vi "DAQNavi Create Channel(Buffered-CI-UpDown Count Value).vi"(0 "task in":i32=-1, 5 "physical channels":string="PCI-1784,BID#0/cntr0", 7 "signal counting type":string(combo)="PulseDirection", 11 "error in (no error)":errorcluster) -> (4 "task out":i32, 15 "error out":errorcluster)   [LabVIEW 2020]
uses:
  DAQNavi_LV.dll
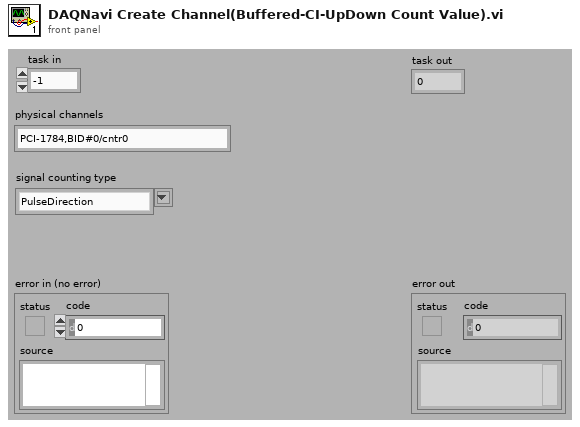
[diagram p1: front panel]
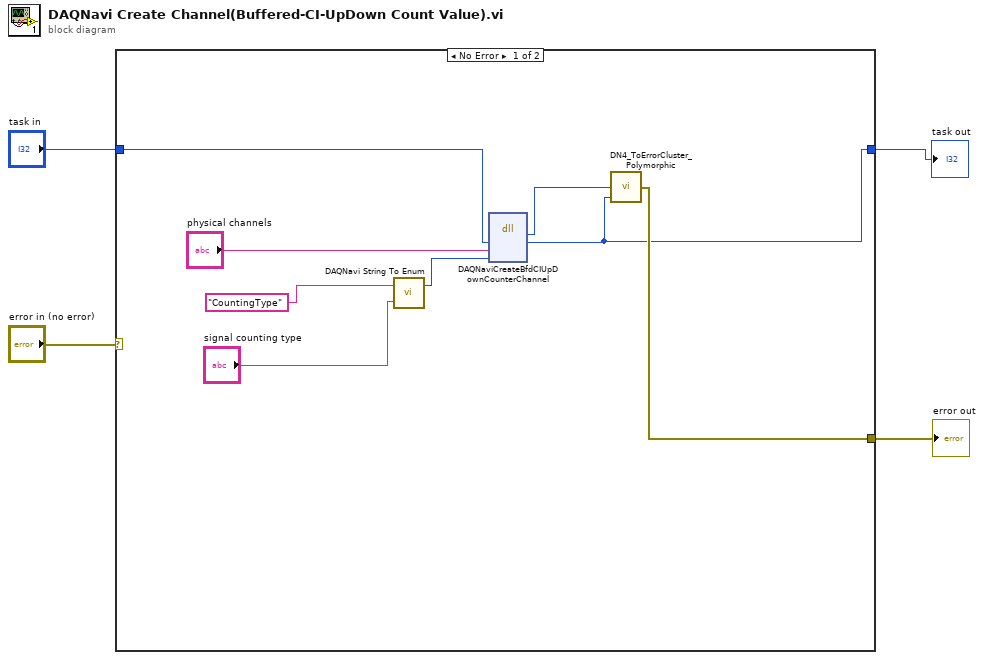
[diagram p0: block diagram]
diagram:
  n1 = case shown="No Error" "error in (no error)" {
    selector: "error in (no error)" -> [_ w13]
    tunnel: [w5 w14] -> w3
    tunnel: "task in" -> [w8 w14]
    tunnel: [w6 w13] -> w1
    frame No Error {
      n2 = call "DAQNavi String To Enum.vi"("enumString"="signal counting type", "enumTypeName"="CountingType") -> ("enumValue"=w10:i32)  [unwired: 1 out]
      n3 = dll-call lib="DAQNavi_LV.dll" fn="DAQNaviCreateBfdCIUpDownCounterChannel"("taskId"=w8, "physicalChannel"="physical channels", "type"=w10) -> ("return type"=w7:i32, "taskId"=w5:i32)  [unwired: 5 in, 2 out]
      n4 = call "DN4_ToErrorCluster_Polymorphic.vi"("task id"=w5, "error code"=w7) -> ("error out"=w6:errorcluster)  [unwired: 3 out]
    }
    frame Error {
    }
  }
  "task out" <- w3
  "error out" <- w1
